vi "Run RealTimeMain.vi"() -> ()   [LabVIEW 2012]
panel:
  in  "Average N Reference Frames":dbl=1.0 min=1.0
  in  "Position Shift Limit (Microns)":dbl=3.0 min=0.0
  out "Out of Limits":bool
  in  "Display Trace Offset (Microns)":dbl=5.0 min=0.0
  in  "output cluster":T1
  out "Z2":dbl[][](graph)=[[-0.26565398159854325, 5.190448689568315]]
  out "Y2":dbl[][](graph)=[[-0.26565398159854325, 5.190448689568315]]
  out "X2":dbl[][](graph)=[[-0.26565398159854325, 5.190448689568315]]
  out "Z1":dbl[][](graph)=[[0.023788275848097486, 4.878801842612402]]
  out "Y1":dbl[][](graph)=[[0.023788275848097486, 4.878801842612402]]
  out "X1":dbl[][](graph)=[[0.023788275848097486, 4.878801842612402]]
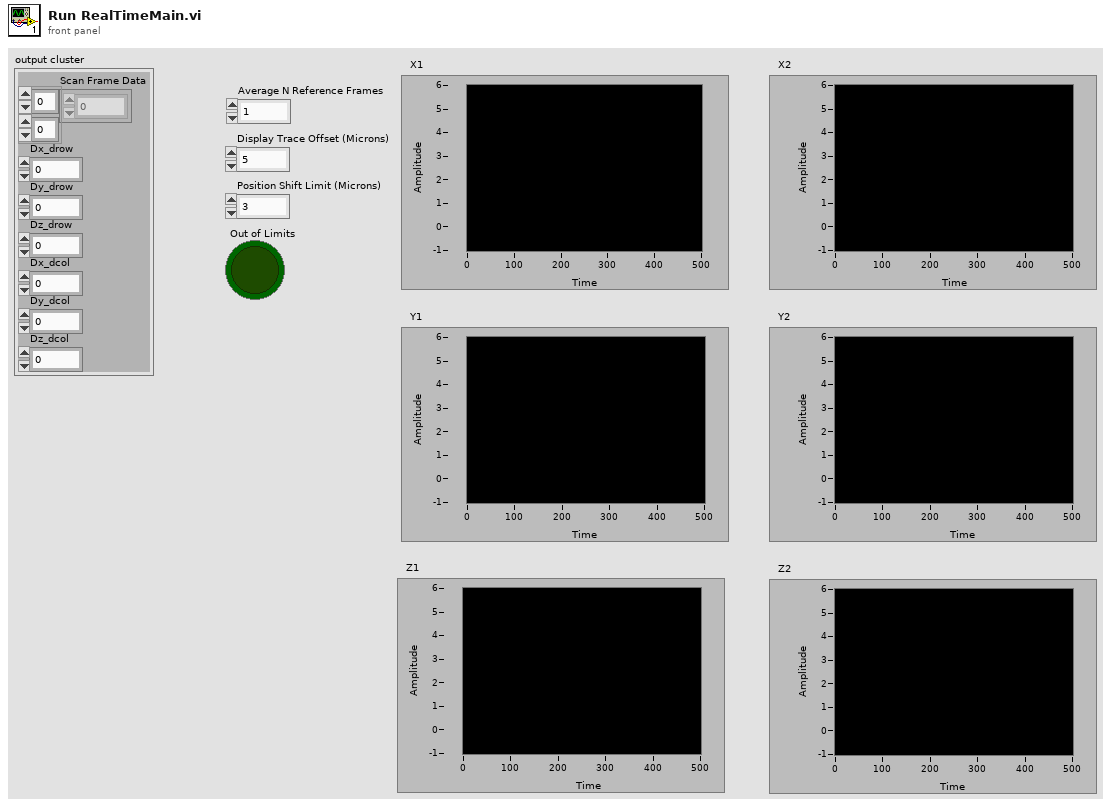
[diagram p1: front panel]
types:
  T1 = cluster{"Scan Frame Data":dbl[][], "Dx_drow":dbl, "Dy_drow":dbl, "Dz_drow":dbl, "Dx_dcol":dbl, "Dy_dcol":dbl, "Dz_dcol":dbl}
  T2 = cluster{"PMTChans":i32, "NumScanPlanes":i32, "ScanRows":i32, "ScanCols":i32, "NumSamples":i32}
  T3 = cluster{"Scan Frame Data":dbl[][], "Dx_drow":dbl, "Dy_drow":dbl, "Dz_drow":dbl, "Dx_dcol":dbl, "Dy_dcol":dbl, "Dz_dcol":dbl}[]
  T4 = cluster{"Scan Frame Data":dbl[][], dbl, dbl, dbl, dbl, dbl, dbl}
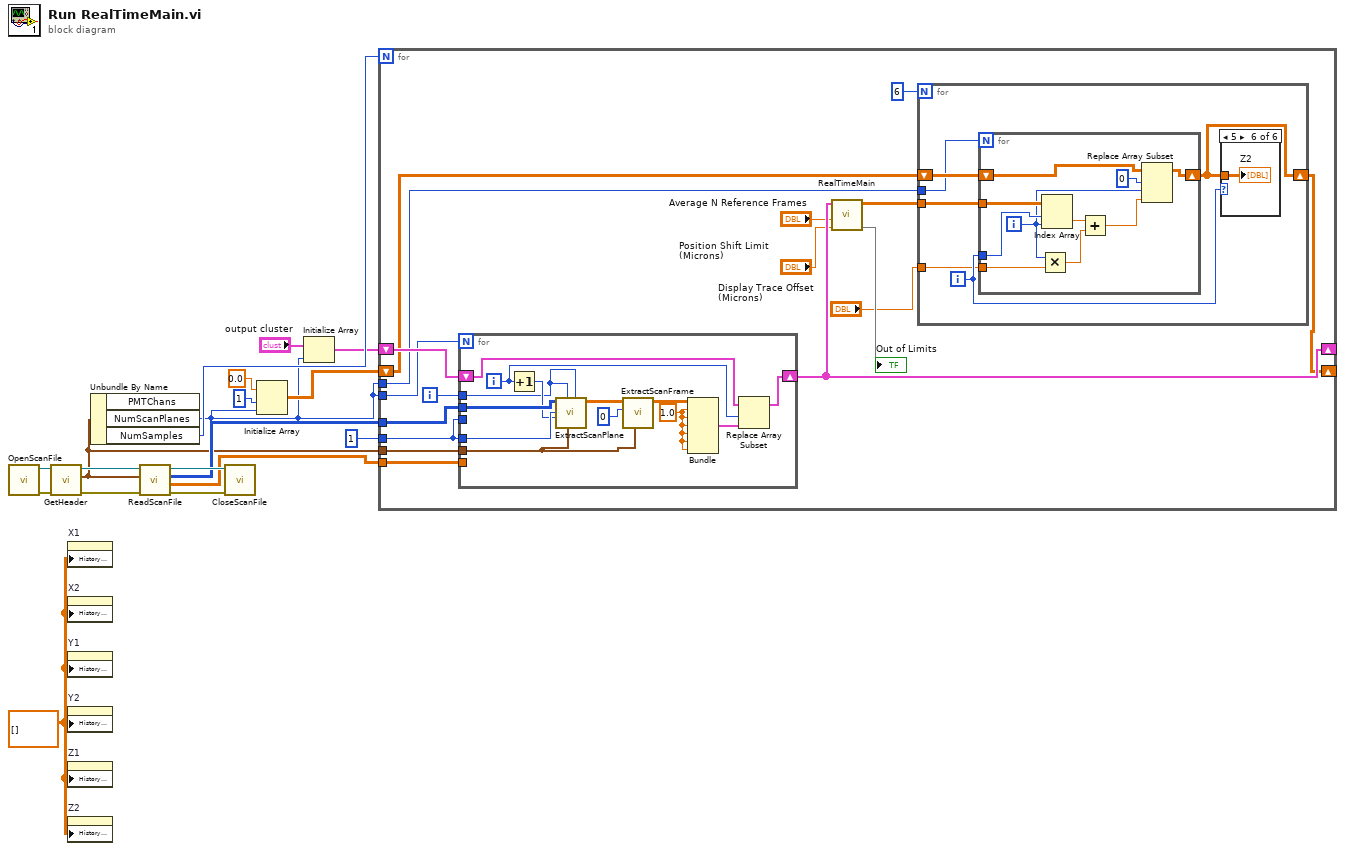
[diagram p0: block diagram]
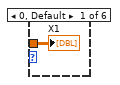
[diagram p2: hidden frame]
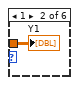
[diagram p3: hidden frame]
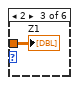
[diagram p4: hidden frame]
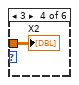
[diagram p5: hidden frame]
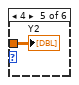
[diagram p6: hidden frame]
diagram:
  w2 = dbl[][] [] ("History Data")
  n1 = call "OpenScanFile.vi"() -> ("error out"=w17:errorcluster, "refnum out"=w18:refnum<file>)  [unwired: 10 in]
  n2 = call "GetHeader.vi"("error in"=w17, "refnum in"=w18) -> ("error out"=w13:errorcluster, "Header"=w10:T2, "refnum out"=w16:refnum<file>)  [unwired: 6 in]
  n3 = property on="X1" class="WFChart (strict)"("History Data"=w2) -> ()  [unwired: 2 in, 2 out]
  n4 = property on="X2" class="WFChart (strict)"("History Data"=w2) -> ()  [unwired: 2 in, 2 out]
  n5 = property on="Y1" class="WFChart (strict)"("History Data"=w2) -> ()  [unwired: 2 in, 2 out]
  n6 = property on="Y2" class="WFChart (strict)"("History Data"=w2) -> ()  [unwired: 2 in, 2 out]
  n7 = property on="Z1" class="WFChart (strict)"("History Data"=w2) -> ()  [unwired: 2 in, 2 out]
  n8 = property on="Z2" class="WFChart (strict)"("History Data"=w2) -> ()  [unwired: 2 in, 2 out]
  n9 = Unbundle By Name(w10) -> ("NumScanPlanes"=w1:i32, "NumSamples"=w8:i32)  [unwired: 1 out]
  n10 = call "ReadScanFile.vi"("error in"=w13, "Header"=w10, "refnum in"=w16) -> ("error out"=w14:errorcluster, "Coordinate Data"=w11:dbl[][][][], "Scan Data"=w12:i32[][][][], "refnum out"=w15:refnum<file>)  [unwired: 5 in]
  n11 = call "CloseScanFile.vi"("error in"=w14, "refnum"=w15) -> ()  [unwired: 9 in, 1 out]
  n12 = Initialize Array(0.0 ("element"), 1 ("dimension size"), w1) -> (w3:dbl[][])
  n13 = Initialize Array("output cluster", w1) -> (w6:T3)
  n14 = for {
    N: w8 -> [_]
    tunnel: w12 -> [w35]
    tunnel: w11 -> [w34]
    tunnel: w10 -> [w33]
    tunnel: w1 -> [w29]
    tunnel: 1 ("x+1") -> [w32]
    shift-right: [w27] -> _
    shift-left: w6 -> [w30]
    tunnel: w1 -> [w21]
    shift-right: [w19] -> _
    shift-left: w3 -> [w28]
    i -> [w31]
    n15 = for {
      N: w29 -> [_]
      tunnel: w35 -> [w70]
      tunnel: w32 -> [w69]
      tunnel: w34 -> [_]
      tunnel: w33 -> [w66]
      tunnel: w32 -> [_]
      tunnel: w31 -> [w60]
      shift-right: [w61] -> w27
      shift-left: w30 -> [w64]
      i -> [w62]
      w58 = 1.0
      n16 = Increment(x=w62) -> (x+1=w67:i32)
      n17 = call "ExtractScanPlane.vi"("End Frame"=w60, "Header"=w66, "Start Frame"=w60, "Scan Plane"=w67, "PMT Channel"=w69, "All Scan Data"=w70) -> ("Scan Plane Data"=w68:dbl[][][])  [unwired: 5 in]
      n18 = call "ExtractScanFrame.vi"("Header"=w66, "Scan Frame"=0, "Scan Plane Data"=w68) -> ("Scan Frame Data"=w65:dbl[][])  [unwired: 8 in]
      n19 = Bundle("Scan Frame Data"=w65, w58, w58, w58, w58, w58, w58) -> (w63:T4)  [unwired: 1 in]
      n20 = Replace Array Subset(array=w64, new element=w63, index=w62) -> (w61:T3)
    }
    n21 = call "RealTimeMain.vi"(8:"Position Shift Limit (Microns)", "For Reference (frames)"="Average N Reference Frames", "Motion Data"=w27) -> (0:→"Out of Limits", "Array"=w26:dbl[][])  [unwired: 7 in]
    n22 = for {
      N: 6 -> [_]
      tunnel: w26 -> [w40]
      tunnel: "Display Trace Offset (Microns)" -> [w37]
      tunnel: w21 -> [w36]
      shift-right: [w38] -> w19
      shift-left: w28 -> [w41]
      i -> [w39]
      n23 = for {
        N: w36 -> [_]
        tunnel: w40 -> [w51]
        tunnel: w39 -> [w50]
        tunnel: w37 -> [w45]
        shift-right: [w47] -> w38
        shift-left: w41 -> [w49]
        i -> [w46]
        n24 = Multiply(x=w46, y=w45) -> (x*y=w44:dbl)
        n25 = Index Array(array=w51, index (row)=w50, index (col)=w46) -> (element=w43:dbl)
        n26 = Add(x=w43, y=w44) -> (x+y=w42:dbl)
        n27 = Replace Array Subset(array=w49, new element=w42, index (row)=0, index (col)=w46) -> (w47:dbl[][])
      }
      n28 = case shown="5" w39 {
        tunnel: w38 -> [w52 w53 w54 w55 w56 w57]
        frame 0, Default {
          "X1" <- w52
        }
        frame 1 {
          "Y1" <- w53
        }
        frame 2 {
          "Z1" <- w54
        }
        frame 3 {
          "X2" <- w55
        }
        frame 4 {
          "Y2" <- w56
        }
        frame 5 {
          "Z2" <- w57
        }
      }
    }
  }
